vi "openbci_read_until_eot.vi"(8 "error in":errorcluster, 10 "EOT_string($$$)":string="$$$", 11 "OBCI dev in":T1={"COM port"="", "n_ch (8)"=enum."8 Channels", "delay_tx"=50}) -> (0 "error out":errorcluster, 2 "string":string, 3 "OBCI dev out":T1={"COM port"="", "n_ch (8)"=enum."8 Channels", "delay_tx"=50})   [LabVIEW 2013]
doc: "Reads Transmission until EOT (EOT) is found"
uses:
  Comm Protocol/Control Def/openbci_device.ctl
  Comm Protocol/Control Def/channel_count.ctl
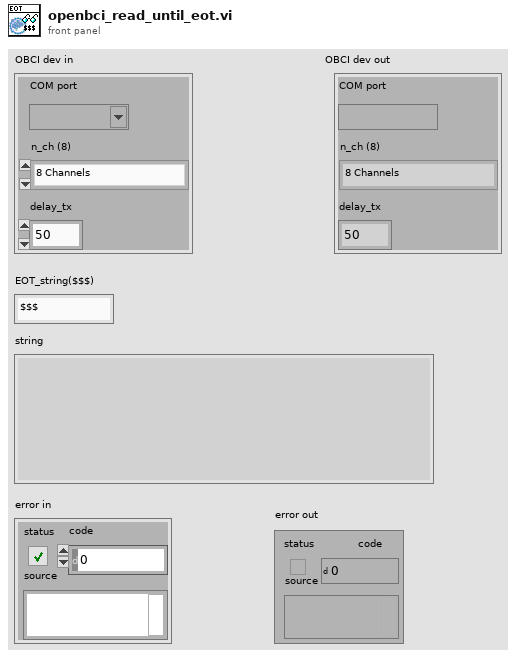
[diagram p1: front panel]
types:
  T1 = typedef "openbci_device.ctl" = cluster{"COM port":refnum<visa-resource-name>, "n_ch (8)":T2, "delay_tx":u32}
  T2 = typedef "channel_count.ctl" = enum16{"8 Channels", "16 Channels"}
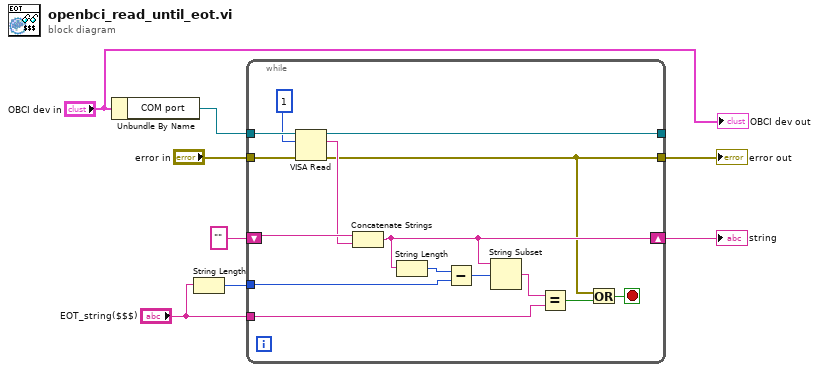
[diagram p0: block diagram]
diagram:
  n1 = Unbundle By Name("OBCI dev in") -> ("COM port"=w2:refnum<visa-resource-name>)
  n2 = String Length(string="EOT_string($$$)") -> (length=w6:i32)
  n3 = while {
    tunnel: w2 -> [w23]
    tunnel: "error in" -> [w22]
    tunnel: [w21] -> _
    shift-right: [w16] -> w4
    shift-left: "" ("read buffer") -> [w18]
    tunnel: w6 -> [w14]
    tunnel: "EOT_string($$$)" -> [w11]
    tunnel: [w9] -> w3
    stop <- w19 stop-if-true
    n4 = VISA Read(VISA resource name=w23, byte count=u32 1, error in (no error)=w22) -> (VISA resource name out=w21:refnum<visa-resource-name>, read buffer=w17:string, error out=w9:errorcluster)  [unwired: 1 out]
    n5 = Concatenate Strings(w18, w17) -> (w16:string)
    n6 = String Length(string=w16) -> (length=w15:i32)
    n7 = Subtract(x=w15, y=w14) -> (x-y=w13:i32)
    n8 = String Subset(string=w16, offset (0)=w13) -> (substring=w12:string)  [unwired: 1 in]
    n9 = Equal?(x=w12, y=w11) -> (x = y?=w10:bool)
    n10 = Or(x=w9, y=w10) -> (x .or. y?=w19:bool)
  }
  "string" <- w4
  "error out" <- w3
  "OBCI dev out" <- "OBCI dev in"
